vi "MB Read Multi Hold Registers.vi"(8 "error in":errorcluster, 11 "Devices":T1) -> (0 "error out":errorcluster, 3 "Register Values":u16[](array[numeric]))   [LabVIEW 2021]
uses:
  <vilib>/NI/Modbus Library/API/Master/Modbus Master.lvclass
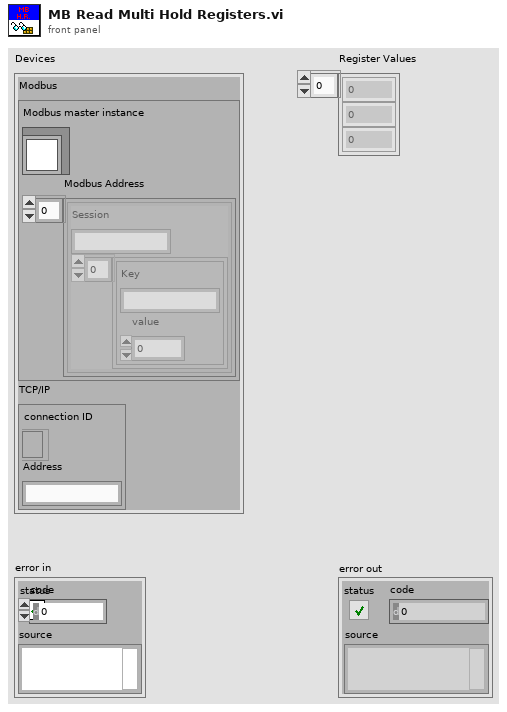
[diagram p1: front panel]
types:
  T1 = cluster{"Modbus":cluster{"Modbus master instance":refnum<class "Modbus Master.lvclass">, "Modbus Address":cluster{"Session":string, cluster{"Key":string, "value":u32}[]}[]}, "TCP/IP":cluster{"connection ID":refnum<k5>, "Address":string}}
  T2 = cluster{"Session":string, cluster{"Key":string, "value":u32}[]}[]
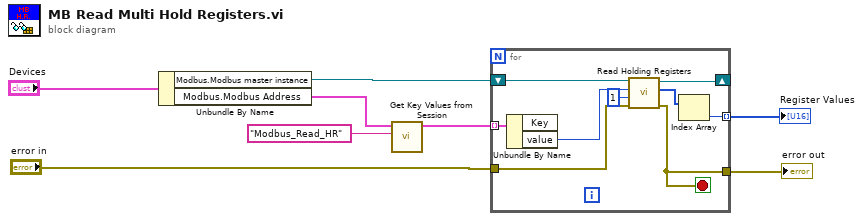
[diagram p0: block diagram]
diagram:
  n1 = Unbundle By Name("Devices") -> ("Modbus.Modbus master instance"=w8:refnum<class "Modbus Master.lvclass">, "Modbus.Modbus Address"=w6:T2)
  n2 = call "Get Key Values from Session.vi"("Session"="Modbus_Read_HR", "Ini File"=w6) -> ("Keys Values in Session"=w4:cluster{"Key":string, "value":u32}[])  [unwired: 7 in, 2 out]
  n3 = for {
    tunnel: w4 -> [w14] mode=indexing
    shift-right: [w16] -> _
    shift-left: w8 -> [w17]
    tunnel: "error in" -> [w15]
    tunnel: [w11] -> w2 mode=indexing
    tunnel: [w10] -> w1
    stop <- w10 stop-if-true
    n4 = Unbundle By Name(w14) -> ("value"=w13:u32)  [unwired: 1 out]
    n5 = call-dynamic "Read Holding Registers.vi"("error in"=w15, "number of inputs"=u16 1, "starting address"=w13, "Modbus master in"=w17) -> ("error out"=w10:errorcluster, "register values"=w12:u16[], "Modbus master out"=w16:refnum<class "Modbus Master.lvclass">)  [unwired: 5 in]
    n6 = Index Array(array=w12) -> (element=w11:u16)  [unwired: 1 in]
  }
  "Register Values" <- w2
  "error out" <- w1
